vi "Add Tool From Dialog.vi"(8 "error in (no error)":errorcluster, 11 "Server Creator Data in":T1) -> (0 "error out":errorcluster, 3 "Server Creator Data out":T1)   [LabVIEW 2025, in "Tools.lvlib"]
uses:
  Tools.lvlib
  Server Creator Data.ctl
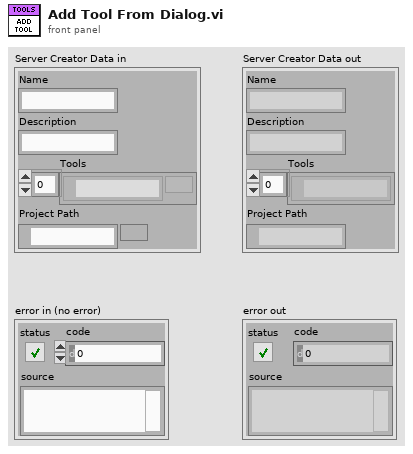
[diagram p1: front panel]
types:
  T1 = typedef "Tools.lvlib/Server Creator Data.ctl" = cluster{"Name":string, "Description":string, "Tools":path[], "Project Path":path}
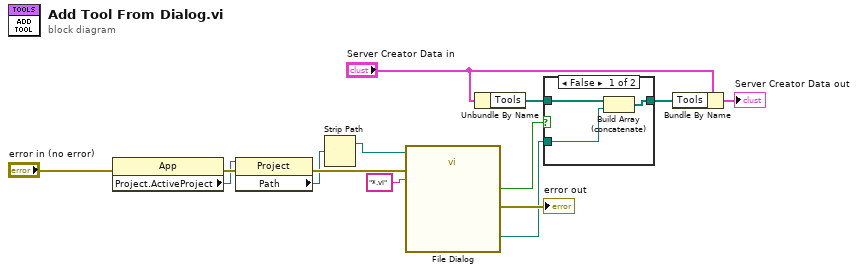
[diagram p0: block diagram]
diagram:
  n1 = property class="App"(error in="error in (no error)") -> (error out=w12:errorcluster, "Project.ActiveProject"=w6:refnum<vi>)  [unwired: 1 in, 1 out]
  n2 = property class="Project"(reference=w6, error in=w12) -> (error out=w13:errorcluster, "Path"=w7:path)  [unwired: 1 out]
  n3 = Strip Path(path=w7) -> (stripped path=w8:path)  [unwired: 1 out]
  n4 = call "File Dialog"("start path"=w8, "error in"=w13, "pattern (all files)"="*.vi" ("pattern label")) -> ("selected path"=w9:path, "cancelled"=w10:bool, "error out"=→"error out":errorcluster)  [unwired: 9 in, 1 out]
  n5 = Unbundle By Name("Server Creator Data in") -> ("Tools"=w3:path[])
  n6 = case shown="False" w10 {
    tunnel: w3 -> [w17 w18]
    tunnel: [w16 w18] -> w4
    tunnel: w9 -> [w15 _]
    frame False {
      n7 = Build Array (concatenate)(w17, w15) -> (w16:path[])
    }
    frame True {
    }
  }
  n8 = Bundle By Name(cluster="Server Creator Data in", "Tools"=w4) -> (→"Server Creator Data out":T1)
